vi "SA_ATTEN.vi"(0 "Session In":refnum<visa-resource-name>="TCPIP0::K-N90X0A-00005.local::inst0::INSTR", 5 "ATT":i32 min=0 max=60 step=10, 11 "error in":errorcluster {"code" format="%.0x"}, 12 "AUTO ATT":i32(ring) items=["OFF", "ON"], 13 "RO(T)":bool, 14 "Timeout":u32=3000) -> (4 "Session Out":refnum<visa-resource-name>, 6 "ATT READ":dbl, 10 "AUTO READ":dbl, 15 "error out":errorcluster {"code" format="%.0x"})   [LabVIEW 2018]
doc: "Launches the Instrument I/O Assistant, which you can use to communicate with message-based instruments and graphically parse the response. For example you can communicate with an instrument that uses a serial, Ethernet, or GPIB interface."
panel:
  in  "Delay Time (s)":dbl=1.0
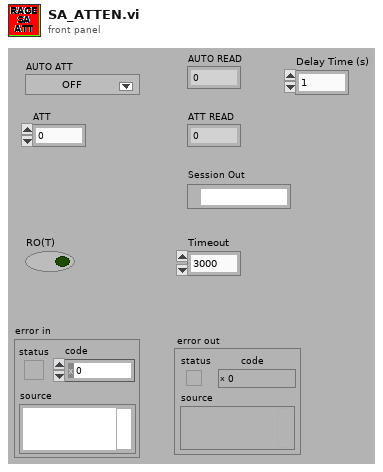
[diagram p1: front panel]
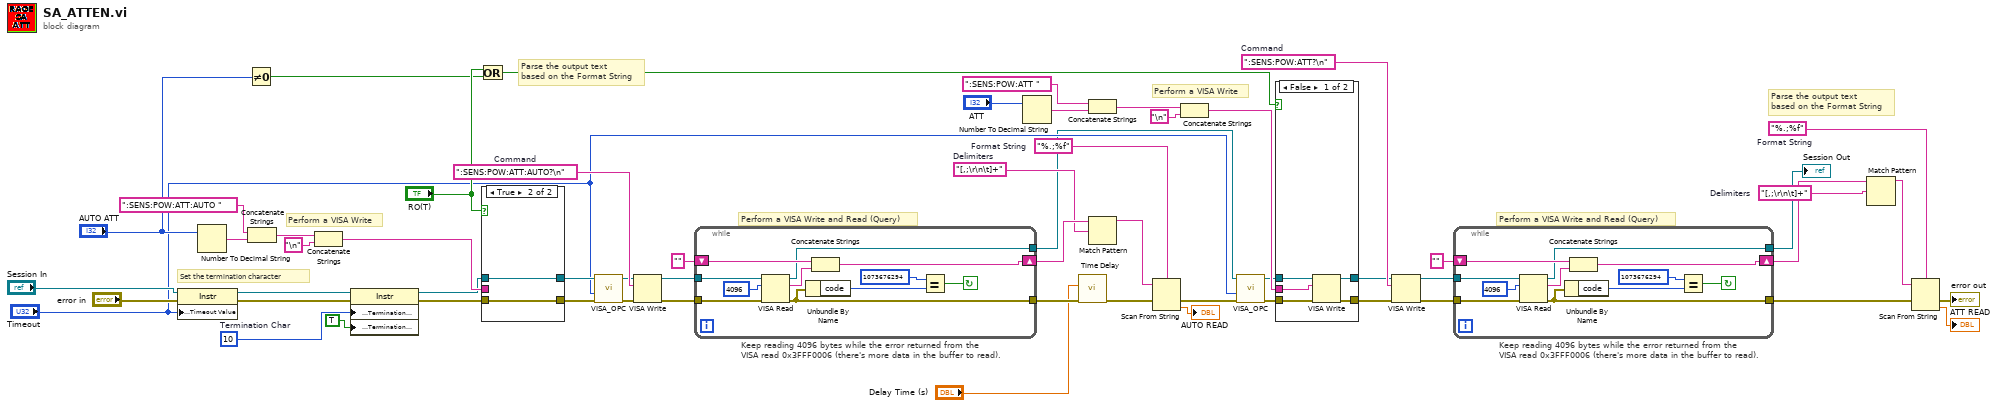
[diagram p0: block diagram]
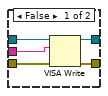
[diagram p3: hidden frame]
diagram:
  w18 = "[,;\r\n\t]+"  # Delimiters
  w21 = "%.;%f"  # Format String
  w24 = ":SENS:POW:ATT?\n"  # Command
  w35 = "[,;\r\n\t]+"  # Delimiters
  w38 = "%.;%f"  # Format String
  w41 = ":SENS:POW:ATT:AUTO?\n"  # Command
  w53 = u8 10  # Termination Char
  # "Parse the output text based on the Format String"
  # "Perform a VISA Write and Read (Query)"
  # "Keep reading 4096 bytes while the error returned from the\nVISA read 0x3FFF0006 (there's more data in the buffer to read)."
  # "Perform a VISA Write"
  # "Parse the output text based on the Format String"
  # "Perform a VISA Write and Read (Query)"
  # "Keep reading 4096 bytes while the error returned from the\nVISA read 0x3FFF0006 (there's more data in the buffer to read)."
  # "Perform a VISA Write"
  # "Set the termination character"
  n1 = property class="Instr"(reference="Session In", error in="error in", "General Settings:Timeout Value"="Timeout") -> (reference out=w52:refnum<visa-resource-name>, error out=w55:errorcluster)
  n2 = Number To Decimal String(number="AUTO ATT") -> (decimal integer string=w50:string)  [unwired: 1 out]
  n3 = Not Equal To 0?(x="AUTO ATT") -> (x != 0?=w14:bool)
  n4 = Concatenate Strings(":SENS:POW:ATT:AUTO " ("staticText"), w50) -> (w47:string)
  n5 = Concatenate Strings(w47, "\n" ("StaticText")) -> (w48:string)
  n6 = property class="Instr"(reference=w52, error in=w55, "Message Based Settings:Termination Character"=w53, "Message Based Settings:Termination Character Enable"=TRUE ("enable")) -> (reference out=w12:refnum<visa-resource-name>, error out=w54:errorcluster)
  n7 = Or(x="RO(T)", y=w14) -> (x .or. y?=w15:bool)
  n8 = case shown="True" "RO(T)" {
    tunnel: w54 -> [w63 w65]
    tunnel: [w62 w65] -> w8
    tunnel: w48 -> [w61 _]
    tunnel: w12 -> [w60 w64]
    tunnel: [w59 w64] -> w10
    frame False {
      n9 = VISA Write(VISA resource name=w60, write buffer=w61, error in (no error)=w63) -> (VISA resource name out=w59:refnum<visa-resource-name>, error out=w62:errorcluster)  [unwired: 1 out]
    }
    frame True {
    }
  }
  n10 = call "VISA_OPC.vi"("error in"=w8, "Timeout"="Timeout", "Session In"=w10) -> ("error out"=w9:errorcluster, "Session Out"=w11:refnum<visa-resource-name>)  [unwired: 6 in, 1 out]
  n11 = VISA Write(VISA resource name=w11, write buffer=w41, error in (no error)=w9) -> (VISA resource name out=w45:refnum<visa-resource-name>, error out=w44:errorcluster)  [unwired: 1 out]
  n12 = while {
    tunnel: w45 -> [w73]
    shift-right: [w67] -> w40
    shift-left: "" -> [w72]
    tunnel: w44 -> [w70]
    tunnel: [w69] -> w43
    tunnel: [w66] -> w6
    stop <- w68 continue-if-true
    n13 = VISA Read(VISA resource name=w73, byte count=u32 4096 ("byte count (0)"), error in (no error)=w70) -> (VISA resource name out=w66:refnum<visa-resource-name>, read buffer=w71:string, error out=w69:errorcluster)  [unwired: 1 out]
    n14 = Unbundle By Name(w69) -> ("code"=w75:i32)
    n15 = Concatenate Strings(w72, w71) -> (w67:string)
    n16 = Equal?(x=1073676294, y=w75) -> (x = y?=w68:bool)
  }
  n17 = Number To Decimal String(number="ATT") -> (decimal integer string=w34:string)  [unwired: 1 out]
  n18 = call "Time Delay"("error in (no error)"=w43, "Delay Time (s)"="Delay Time (s)") -> ("error out"=w2:errorcluster)  [unwired: 9 in]
  n19 = Concatenate Strings(":SENS:POW:ATT " ("staticText"), w34) -> (w30:string)
  n20 = Match Pattern(string=w40, regular expression=w35) -> (before substring=w39:string)  [unwired: 1 in, 3 out]
  n21 = Scan From String(format string=w38, input string=w39, error in=w2) -> (error out=w37:errorcluster, output 1=→"AUTO READ":dbl)  [unwired: 2 in, 2 out]
  n22 = Concatenate Strings(w30, "\n" ("StaticText")) -> (w31:string)
  n23 = call "VISA_OPC.vi"("error in"=w37, "Timeout"="Timeout", "Session In"=w6) -> ("error out"=w13:errorcluster, "Session Out"=w5:refnum<visa-resource-name>)  [unwired: 6 in, 1 out]
  n24 = case shown="False" w15 {
    tunnel: w13 -> [w81 w83]
    tunnel: [w80 w83] -> w32
    tunnel: w31 -> [w79 _]
    tunnel: w5 -> [w78 w82]
    tunnel: [w77 w82] -> w4
    frame False {
      n25 = VISA Write(VISA resource name=w78, write buffer=w79, error in (no error)=w81) -> (VISA resource name out=w77:refnum<visa-resource-name>, error out=w80:errorcluster)  [unwired: 1 out]
    }
    frame True {
    }
  }
  n26 = VISA Write(VISA resource name=w4, write buffer=w24, error in (no error)=w32) -> (VISA resource name out=w28:refnum<visa-resource-name>, error out=w27:errorcluster)  [unwired: 1 out]
  n27 = while {
    tunnel: w28 -> [w91]
    shift-right: [w85] -> w23
    shift-left: "" -> [w90]
    tunnel: w27 -> [w88]
    tunnel: [w87] -> w26
    tunnel: [w84] -> w3
    stop <- w86 continue-if-true
    n28 = VISA Read(VISA resource name=w91, byte count=u32 4096 ("byte count (0)"), error in (no error)=w88) -> (VISA resource name out=w84:refnum<visa-resource-name>, read buffer=w89:string, error out=w87:errorcluster)  [unwired: 1 out]
    n29 = Unbundle By Name(w87) -> ("code"=w93:i32)
    n30 = Concatenate Strings(w90, w89) -> (w85:string)
    n31 = Equal?(x=1073676294, y=w93) -> (x = y?=w86:bool)
  }
  "Session Out" <- w3
  n32 = Match Pattern(string=w23, regular expression=w18) -> (before substring=w22:string)  [unwired: 1 in, 3 out]
  n33 = Scan From String(format string=w21, input string=w22, error in=w26) -> (error out=→"error out":errorcluster, output 1=→"ATT READ":dbl)  [unwired: 2 in, 2 out]
